vi "Update Message.vi"(8 "error in (no error)":errorcluster, 10 "Message":string, 11 "Chat Window Panel in":refnum<class "Chat Window Panel.lvclass">) -> (0 "error out":errorcluster, 3 "Chat Window Panel out":refnum<class "Chat Window Panel.lvclass">)   [LabVIEW 2018, in "Chat Window Panel.lvlib" / "Chat Window Panel.lvclass"]
uses:
  Chat Window Panel.lvclass
  Chat Window Panel.lvclass/Chat Window Panel.ctl
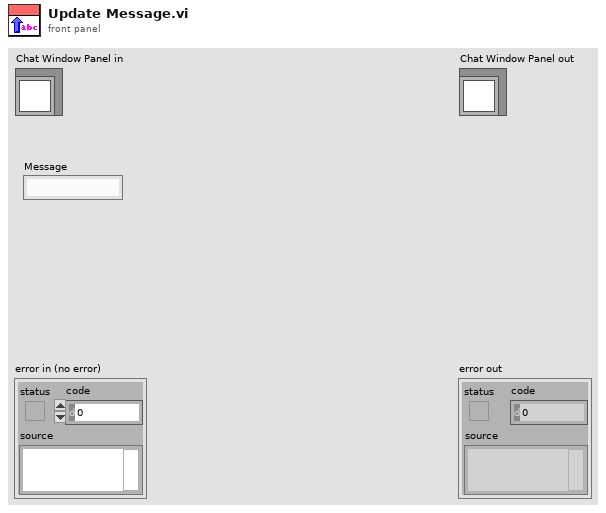
[diagram p1: front panel]
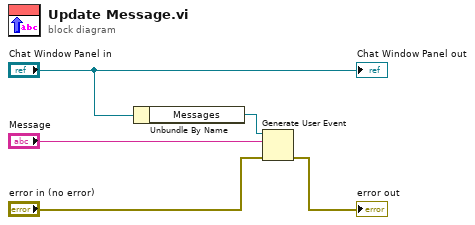
[diagram p0: block diagram]
diagram:
  n1 = Unbundle By Name("Chat Window Panel in") -> ("Messages"=w4:refnum<user-event>)
  n2 = Generate User Event(user event=w4, event data cluster="Message", error in="error in (no error)") -> (error out=→"error out":errorcluster)  [unwired: 1 in, 1 out]
  "Chat Window Panel out" <- "Chat Window Panel in"
